vi "JLINKARM Go Ex.vi"(8 "error in (no error)":errorcluster caption="错误输入（无错误）", 10 "param2":i32, 11 "param1":i32) -> (0 "error out":errorcluster caption="错误输出", 3 "function return":i32)   [LabVIEW 2016, in "JLinkARM.lvlib"]
doc: "int JLINKARM_GoEx(int param1, int param2);"
uses:
  <userlib>/LV-JLinkARM/JLinkARM.lvlib
  <userlib>/LV-JLinkARM/JLinkARM.dll
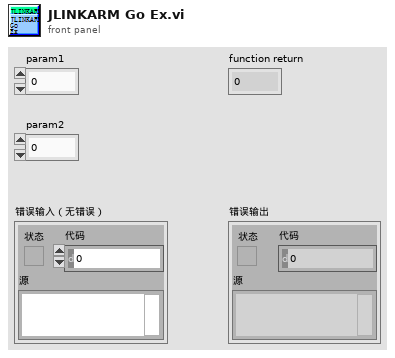
[diagram p1: front panel]
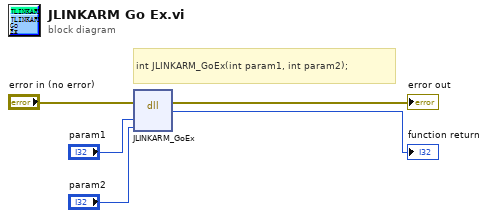
[diagram p0: block diagram]
diagram:
  # "int JLINKARM_GoEx(int param1, int param2);"
  n1 = dll-call lib="C:/Program Files (x86)/National Instruments/LabVIEW 2016/user.lib/LV-JLinkARM/JLinkARM.*" fn="JLINKARM_GoEx"(error in="error in (no error)", "param1"="param1", "param2"="param2") -> (error out=→"error out":errorcluster, →"function return":i32)  [unwired: 4 in, 1 out]
